vi "Unpack message frame.vi"(8 "error in":errorcluster, 11 "Message frame":u8[](array[numeric])) -> (0 "error IO":errorcluster, 1 "Size (bytes)":i32, 2 "Message Type":T1)   [LabVIEW 2020, in "wamplv.lvlib" / "RawSocket Handler.lvclass"]
uses:
  RawSocket Handler.lvclass
  Message Type.ctl
  <vilib>/Utility/error.llb/Error Cluster From Error Code.vi
  <vilib>/ErrorRing/Error Ring.xnode
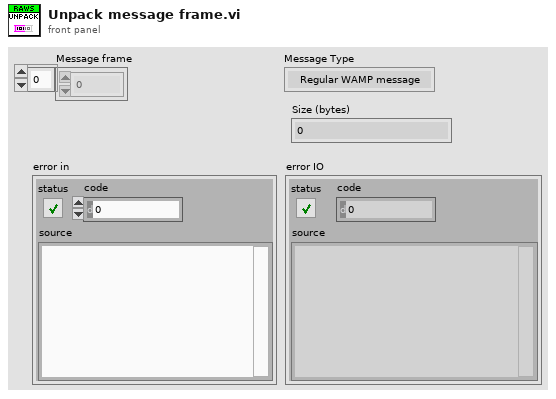
[diagram p1: front panel]
types:
  T1 = typedef "wamplv.lvlib/RawSocket Handler.lvclass/Message Type.ctl" = enum8{"Regular WAMP message", "PING", "PONG"}
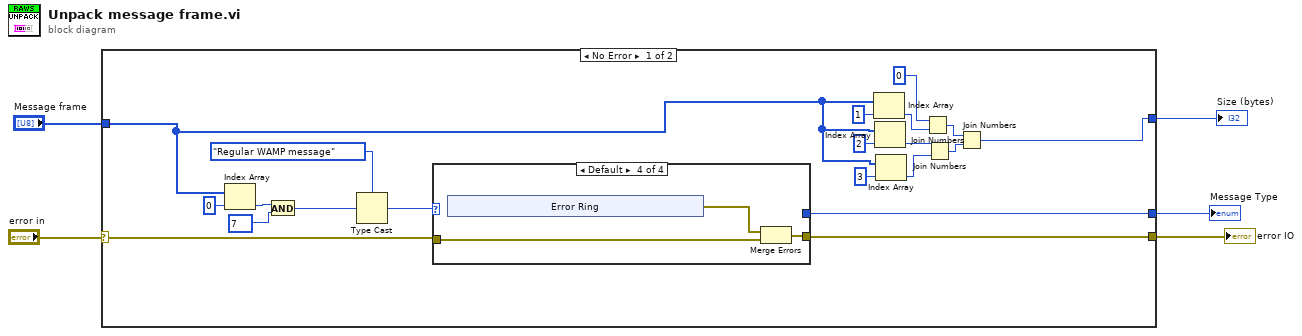
[diagram p0: block diagram]
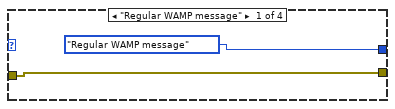
[diagram p2: hidden frame]
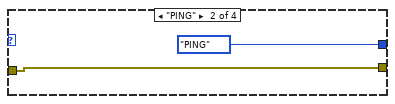
[diagram p3: hidden frame]
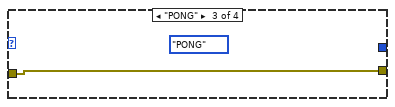
[diagram p4: hidden frame]
diagram:
  n1 = case shown="No Error" "error in" {
    selector: "error in" -> [w25 w38]
    tunnel: "Message frame" -> [w13 _]
    tunnel: [w7 _] -> w3
    tunnel: [w21 w38] -> w2
    tunnel: [w17 _] -> w1
    frame No Error {
      n2 = Index Array(array=w13, index=0) -> (element=w23:u8)
      n3 = And(x=w23, y=u8 7) -> (x .and. y?=w20:u8)
      n4 = Type Cast(type=Message_Type."Regular WAMP message" ("Message Type"), x=w20) -> (*(type *) &x=w18:T1)
      n5 = case shown="Default" w18 {
        tunnel: w25 -> [w27 w29 w30 w33]
        tunnel: [w27 w29 w30 w32] -> w21
        tunnel: [Message_Type."Regular WAMP message" ("Message Type") Message_Type."PING" ("Message Type") _ _] -> w17
        frame "Regular WAMP message" {
        }
        frame "PING" {
        }
        frame "PONG" {
          (unwired) Message_Type."PONG" ("Message Type")
        }
        frame Default {
          n6 = xnode "Error Ring"() -> ("error out"=w31:errorcluster)
          n7 = Merge Errors(w31, w33) -> (w32:errorcluster)
        }
      }
      n8 = Index Array(array=w13, index=1) -> (element=w12:u8)
      n9 = Index Array(array=w13, index=2) -> (element=w10:u8)
      n10 = Index Array(array=w13, index=3) -> (element=w11:u8)
      n11 = Join Numbers(hi=u8 0, lo=w12) -> ((hi.lo)=w9:u16)
      n12 = Join Numbers(hi=w10, lo=w11) -> ((hi.lo)=w8:u16)
      n13 = Join Numbers(hi=w9, lo=w8) -> ((hi.lo)=w7:u32)
    }
    frame Error {
    }
  }
  "Message Type" <- w1
  "Size (bytes)" <- w3
  "error IO" <- w2
